vi "sub_save-data.vi"(7 "cmd":enum16{"create", "save"}(ring), 8 "error in":errorcluster caption="에러 입력(에러 없음)", 11 "data":string) -> (0 "error out":errorcluster caption="에러 출력")   [LabVIEW 2016]
uses:
  ctl/file_path-cmd.ctl
panel:
  out "appended path":path
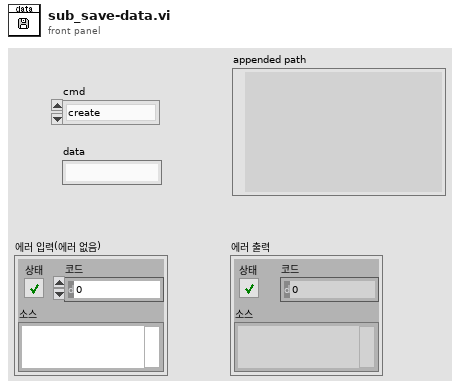
[diagram p1: front panel]
types:
  T1 = typedef "file_path-cmd.ctl" = enum16{"default", "write"}
  T2 = enum16{"open", "replace", "create", "open or create", "replace or create", "replace or create with confirmation"}
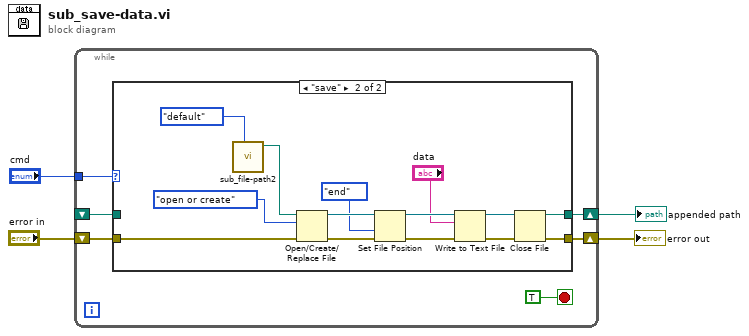
[diagram p0: block diagram]
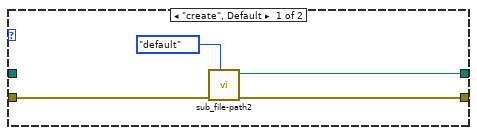
[diagram p2: hidden frame]
diagram:
  n1 = while {
    tunnel: "cmd" -> [w10]
    shift-right: [w7] -> w2
    shift-left: "error in" -> [w8]
    shift-right: [w6] -> w1
    shift-left: _ -> [w5]
    stop <- TRUE stop-if-true
    n2 = case shown="\"save\"" w10 {
      tunnel: w8 -> [w13 w20]
      tunnel: [w12 w19] -> w7
      tunnel: [w11 w17] -> w6
      tunnel: w5 -> [_ _]
      frame "create", Default {
        n3 = call "sub_file-path2.vi"("cmd"=file_path-cmd."default", "error in"=w13) -> ("error out"=w12:errorcluster, "result path"=w11:path)  [unwired: 7 in, 1 out]
      }
      frame "save" {
        n4 = call "sub_file-path2.vi"("cmd"=file_path-cmd."default") -> ("result path"=w16:path)  [unwired: 8 in, 2 out]
        n5 = Open/Create/Replace File(file path (use dialog)=w16, error in=w20, operation (0:open)=T2."open or create" ("동작(0:open)")) -> (refnum out=w23:refnum<file>, error out=w25:errorcluster)  [unwired: 3 in, 1 out]
        n6 = Set File Position(refnum=w23, from (0:start)=enum16{"start", "end", "current"}."end" ("시작(0:시작)"), error in=w25) -> (refnum out=w22:refnum<file>, error out=w24:errorcluster)  [unwired: 1 in]
        n7 = Write to Text File(file (use dialog)=w22, text="data", error in=w24) -> (refnum out=w27:refnum<file>, error out=w28:errorcluster)  [unwired: 1 in, 1 out]
        n8 = Close File(refnum=w27, error in=w28) -> (path=w17:path, error out=w19:errorcluster)
      }
    }
  }
  "error out" <- w2
  "appended path" <- w1
